vi "Plot_Values_Global.vi"() -> ()   [LabVIEW 2018]
panel:
  in  "XY Graph Cluster":cluster{dbl[], dbl[]}[](array[cluster]) {"?" format="%.2f"; "?" format="%.2f"}
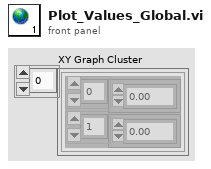
[diagram p1: front panel]
diagram:
